vi "Lookup Configured Group.vi"(8 "error in (no error)":errorcluster, 11 "DataProcessor in":refnum<class "DataProcessor.lvclass">) -> (0 "error out":errorcluster, 3 "DataProcessor out":refnum<class "DataProcessor.lvclass">)   [LabVIEW 2020, in "Volatus.lvlib" / "DataProcessor.lvclass"]
uses:
  DataProcessor.lvclass
  C:/dev/lv20CE/relink/lv-volatus/Volatus/Task/Task.lvclass
  lv-vecto/Vecto/Group/Group.lvclass
  C:/dev/lv20CE/relink/lv-vecto/Vecto/GroupAbstract/GroupAbstract.lvclass
  DataProcessor.lvclass/DataProcessor.ctl
  VolatusConfig/VolatusConfigElement/VolatusConfigElement.lvclass/VolatusConfigElement.ctl
  Task/Task.lvclass/Task.ctl
  TelemetryAPI/TelemetryAPI.lvclass/TelemetryAPI.ctl
  VolatusConfig/VolatusConfigElement/Element.vi
  VolatusConfig/VolatusConfigElement/Lookup Child by Name.vi
  VolatusConfig/Group/Group.lvclass
  C:/dev/lv20CE/relink/lv-volatus/VolatusConfig/VolatusConfigElement/VolatusConfigElement.lvclass
  lv-cdm/CDM-Config/Config Element/Lookup Child by Name.vi
  Task/Task.lvclass
  VolatusConfig/VolatusConfigElement/VolatusConfigElement.lvclass
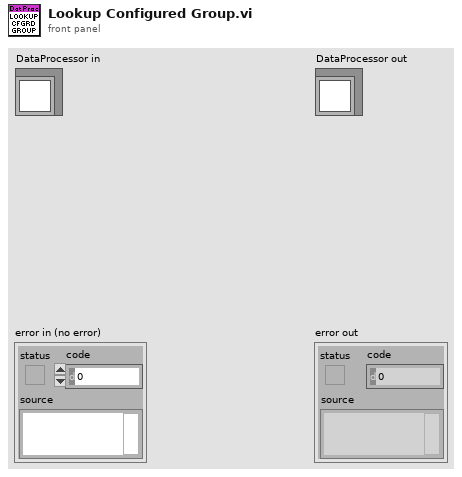
[diagram p1: front panel]
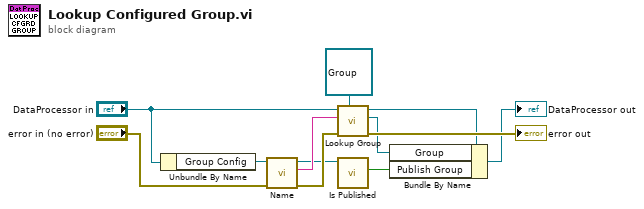
[diagram p0: block diagram]
diagram:
  n1 = Unbundle By Name("DataProcessor in") -> ("Group Config"=w9:refnum<class "Group.lvclass">)
  n2 = call "Name.vi"("error in (no error)"="error in (no error)", "VolatusConfigElement in"=w9) -> ("error out"=w7:errorcluster, "Name"=w8:string, "VolatusConfigElement out"=w2:refnum<class "Group.lvclass">)  [unwired: 7 in]
  n3 = call "Lookup Group.vi"("Group Type (Abstract)"=refnum<class "Group.lvclass"> refnum ("Vecto.lvlib:Group.lvclass"), "error in (no error)"=w7, "Group Name"=w8, "Task in"="DataProcessor in") -> ("error out"=→"error out":errorcluster, "Group"=w5:refnum<class "Group.lvclass">, "Task out"=w10:refnum<class "DataProcessor.lvclass">)  [unwired: 5 in]
  n4 = call "Is Published.vi"("Group in"=w2) -> ("Is Published"=w1:bool)  [unwired: 8 in, 2 out]
  n5 = Bundle By Name(cluster=w10, "Group"=w5, "Publish Group"=w1) -> (→"DataProcessor out":refnum<class "DataProcessor.lvclass">)
